vi "oax_UpdateExtractListBox.vi"(7 "operation":T1(ring), 8 "error in (no error)":errorcluster, 10 "Order to extract":dbl[](array[numeric]), 11 "ref in":refnum<vi>) -> (0 "error out":errorcluster, 2 "orders to extract out":dbl[](array[numeric]), 3 "ref out":refnum<vi>)   [LabVIEW 2017]
uses:
  <vilib>/addons/Sound and Vibration/Order Analysis/Gabor Order Tracking/SoundVib_Gabor.lvlib
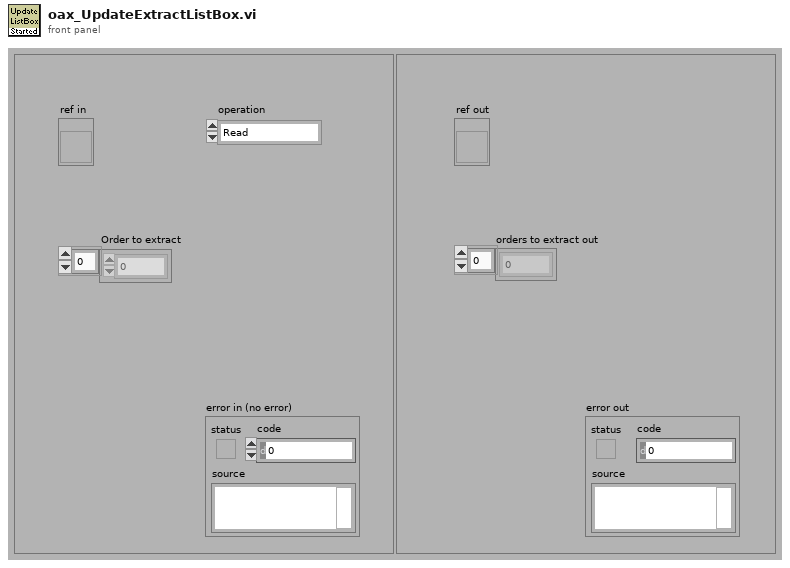
[diagram p1: front panel]
types:
  T1 = enum16{"Read", "Add", "Delete", "Clear", "GetSelected"}
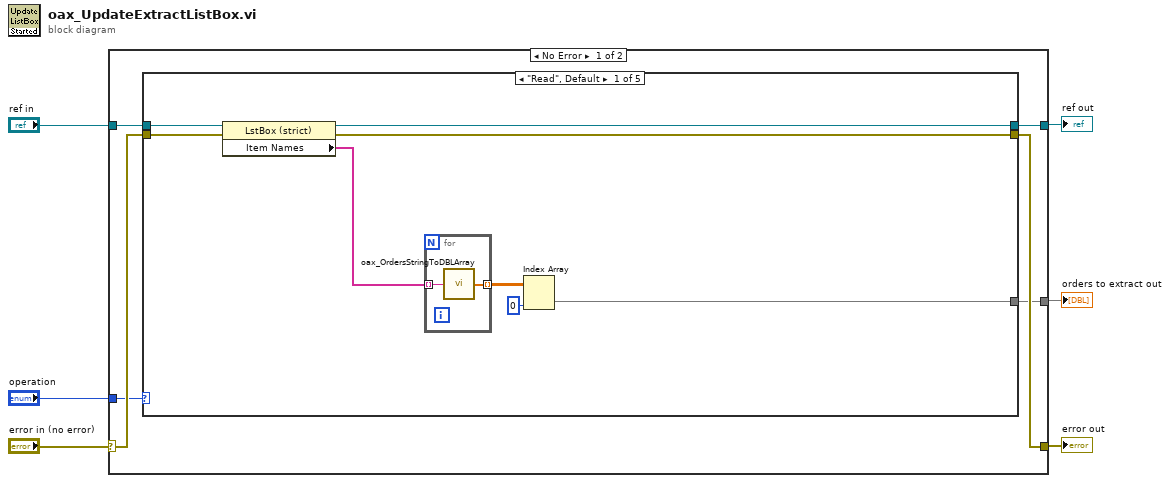
[diagram p0: block diagram]
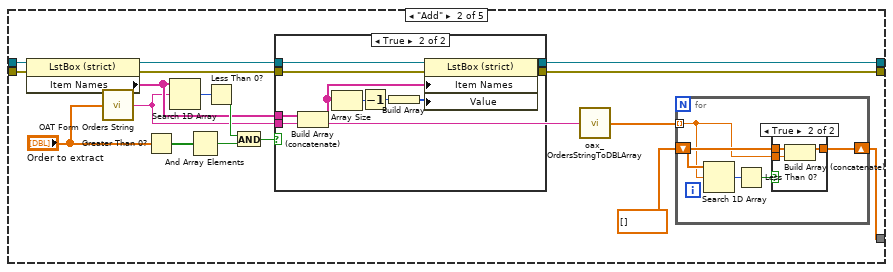
[diagram p2: hidden frame]
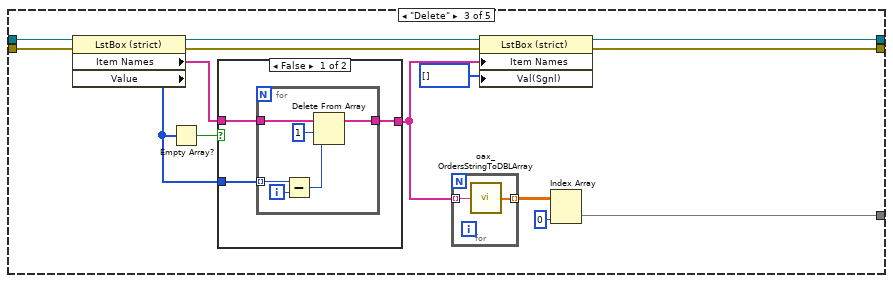
[diagram p5: hidden frame]
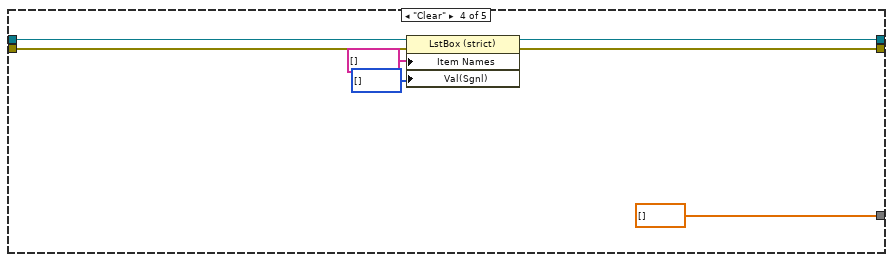
[diagram p7: hidden frame]
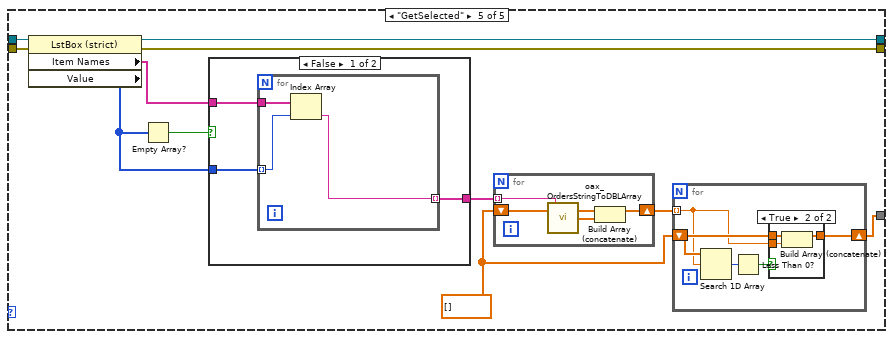
[diagram p8: hidden frame]
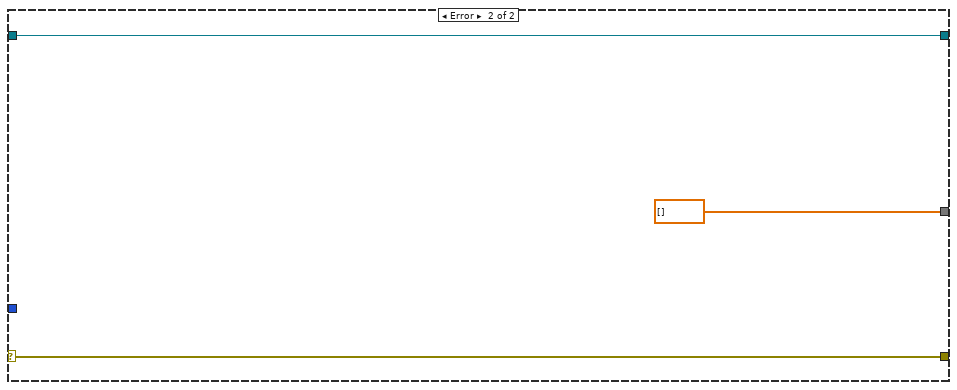
[diagram p11: hidden frame]
diagram:
  n1 = case shown="No Error" "error in (no error)" {
    selector: "error in (no error)" -> [w11 w127]
    tunnel: [w10 w127] -> w5
    tunnel: "ref in" -> [w12 w126]
    tunnel: [w9 w126] -> w3
    tunnel: [w8 dbl[] [] ("orders to extract out")] -> w2
    tunnel: "operation" -> [w7 _]
    frame No Error {
      n2 = case shown="\"Read\", Default" w7 {
        tunnel: w12 -> [w19 w38 w68 w91 w104]
        tunnel: w11 -> [w13 w39 w69 w90 w103]
        tunnel: [w16 w32 w67 w93 w101] -> w10
        tunnel: [w15 w31 w65 w92 w100] -> w9
        tunnel: [w14 w23 w61 dbl[] [] ("orders to extract out") w94] -> w8
        frame "Read", Default {
          n3 = property on="Property Node" class="LstBox (strict)"(reference=w19, error in=w13) -> (reference out=w15:refnum<vi>, error out=w16:errorcluster, "Item Names"=w18:string[])
          n4 = for {
            tunnel: w18 -> [w22] mode=indexing
            tunnel: [w21] -> w17 mode=indexing
            n5 = call <vilib>:"oax_OrdersStringToDBLArray.vi"("orders to extract"=w22) -> ("orders to extract out"=w21:dbl[])
          }
          n6 = Index Array(array=w17, index (col)=0 ("disabled index (col)")) -> (element=w14:dbl[])  [unwired: 1 in]
        }
        frame "Add" {
          n7 = property on="Property Node" class="LstBox (strict)"(reference=w38, error in=w39) -> (reference out=w34:refnum<vi>, error out=w33:errorcluster, "Item Names"=w30:string[])
          n8 = call <vilib>:"OAT Form Orders String.vi"("orders to extract in"="Order to extract") -> ("orders to extract out"=w24:string)
          n9 = Greater Than 0?(x="Order to extract") -> (x > 0?=w28:bool[])
          n10 = Search 1D Array(1D array=w30, element=w24) -> (index of element=w37:i32)  [unwired: 1 in]
          n11 = And Array Elements(Boolean array=w28) -> (logical AND=w27:bool)
          n12 = Less Than 0?(x=w37) -> (x < 0?=w36:bool)
          n13 = And(x=w36, y=w27) -> (x .and. y?=w35:bool)
          n14 = case shown="True" w35 {
            tunnel: w34 -> [w49 w58]
            tunnel: w33 -> [w50 w59]
            tunnel: [w50 w56] -> w32
            tunnel: [w49 w57] -> w31
            tunnel: w24 -> [_ w51]
            tunnel: w30 -> [_ w60]
            frame False {
            }
            frame True {
              n15 = Build Array (concatenate)(w60, w51) -> (w55:string[])
              n16 = Array Size(array=w55) -> (size(s)=w54:i32)
              n17 = Decrement(x=w54) -> (x-1=w52:i32)
              n18 = Build Array(w52) -> (w53:i32[])
              n19 = property on="Property Node" class="LstBox (strict)"(reference=w58, error in=w59, "Item Names"=w55, "Value"=w53) -> (reference out=w57:refnum<vi>, error out=w56:errorcluster)
            }
          }
          n20 = call <vilib>:"oax_OrdersStringToDBLArray.vi"("orders to extract"=w24) -> ("orders to extract out"=w25:dbl[])
          n21 = for {
            tunnel: w25 -> [w41] mode=indexing
            shift-right: [w40] -> w23
            shift-left: dbl[] [] -> [w42]
            n22 = Search 1D Array(1D array=w42, element=w41) -> (index of element=w44:i32)  [unwired: 1 in]
            n23 = Less Than 0?(x=w44) -> (x < 0?=w43:bool)
            n24 = case shown="True" w43 {
              tunnel: w42 -> [w45 w48]
              tunnel: w41 -> [_ w47]
              tunnel: [w45 w46] -> w40
              frame False {
              }
              frame True {
                n25 = Build Array (concatenate)(w48, w47) -> (w46:dbl[])
              }
            }
          }
        }
        frame "Delete" {
          n26 = property on="Property Node" class="LstBox (strict)"(reference=w68, error in=w69) -> (reference out=w66:refnum<vi>, error out=w71:errorcluster, "Item Names"=w72:string[], "Value"=w73:i32[])
          n27 = Empty Array?(array=w73) -> (empty?=w74:bool)
          n28 = case shown="False" w74 {
            tunnel: w73 -> [w79 _]
            tunnel: w72 -> [w78 w86]
            tunnel: [w77 w86] -> w62
            frame False {
              n29 = for {
                tunnel: w79 -> [w82] mode=indexing
                tunnel: w78 -> [w85]
                tunnel: [w80] -> w77
                i -> [w83]
                n30 = Subtract(x=w82, y=w83) -> (x-y=w81:i32)
                n31 = Delete From Array(array=w85, length=1, index=w81) -> (array with subset deleted=w80:string[])  [unwired: 1 out]
              }
            }
            frame True {
            }
          }
          n32 = for {
            tunnel: w62 -> [w76] mode=indexing
            tunnel: [w75] -> w63 mode=indexing
            n33 = call <vilib>:"oax_OrdersStringToDBLArray.vi"("orders to extract"=w76) -> ("orders to extract out"=w75:dbl[])
          }
          n34 = property on="Property Node" class="LstBox (strict)"(reference=w66, error in=w71, "Item Names"=w62, "Val(Sgnl)"=i32[] [] ("Value (Signaling)")) -> (reference out=w65:refnum<vi>, error out=w67:errorcluster)
          n35 = Index Array(array=w63, index (col)=0 ("disabled index (col)")) -> (element=w61:dbl[])  [unwired: 1 in]
        }
        frame "Clear" {
          n36 = property on="Property Node" class="LstBox (strict)"(reference=w91, error in=w90, "Item Names"=string[] [], "Val(Sgnl)"=i32[] [] ("Value (Signaling)")) -> (reference out=w92:refnum<vi>, error out=w93:errorcluster)
        }
        frame "GetSelected" {
          w95 = dbl[] []
          n37 = property on="Property Node" class="LstBox (strict)"(reference=w104, error in=w103) -> (reference out=w100:refnum<vi>, error out=w101:errorcluster, "Item Names"=w99:string[], "Value"=w97:i32[])
          n38 = Empty Array?(array=w97) -> (empty?=w102:bool)
          n39 = case shown="False" w102 {
            tunnel: w99 -> [w120 w124]
            tunnel: [w118 w124] -> w98
            tunnel: w97 -> [w119 _]
            frame False {
              n40 = for {
                tunnel: w120 -> [w123]
                tunnel: w119 -> [w122] mode=indexing
                tunnel: [w121] -> w118 mode=indexing
                n41 = Index Array(array=w123, index=w122) -> (element=w121:string)
              }
            }
            frame True {
            }
          }
          n42 = for {
            tunnel: w98 -> [w117] mode=indexing
            shift-right: [w116] -> w96
            shift-left: w95 -> [w114]
            n43 = call <vilib>:"oax_OrdersStringToDBLArray.vi"("orders to extract"=w117) -> ("orders to extract out"=w115:dbl[])
            n44 = Build Array (concatenate)(w114, w115) -> (w116:dbl[])
          }
          n45 = for {
            tunnel: w96 -> [w106] mode=indexing
            shift-right: [w105] -> w94
            shift-left: w95 -> [w107]
            n46 = Search 1D Array(1D array=w107, element=w106) -> (index of element=w109:i32)  [unwired: 1 in]
            n47 = Less Than 0?(x=w109) -> (x < 0?=w108:bool)
            n48 = case shown="True" w108 {
              tunnel: w107 -> [w110 w113]
              tunnel: w106 -> [_ w112]
              tunnel: [w110 w111] -> w105
              frame False {
              }
              frame True {
                n49 = Build Array (concatenate)(w113, w112) -> (w111:dbl[])
              }
            }
          }
        }
      }
    }
    frame Error {
    }
  }
  "error out" <- w5
  "ref out" <- w3
  "orders to extract out" <- w2
